vi "Test for renamed Wfms.vi"(4 "Full Path info":bool, 6 "Refresh List":bool, 8 "Error In":errorcluster, 9 "ListBox Variant":variant, 10 "CD Settings":T1={"CD Task Dependency"=18446744073709551615, "CD Task Dependency Ref"=18446744073709551615, "CD Task Available Wfms"=[], "CD Task Selected Wfms"=[], "Buffer Length (samples)"=0, "Min Enabled"=FALSE, "Max Enabled "=FALSE, "SP Enabled"=FALSE, "RMS Enabled"=FALSE, "Buffer Length (s)"=0.0, "Task Rate"=0.0, "Number of DAQ Chanels"=0} {"CD Task Dependency Ref" format="%.0x"; "CD Task Dependency" format="%.0x"}, 11 "CustomDevice Ref":T2 format="%.0x") -> (0 "Error Out":errorcluster, 1 "ListBox Variant":variant, 2 "CD Settings out":T1={"CD Task Dependency"=18446744073709551615, "CD Task Dependency Ref"=18446744073709551615, "CD Task Available Wfms"=[], "CD Task Selected Wfms"=[], "Buffer Length (samples)"=0, "Min Enabled"=FALSE, "Max Enabled "=FALSE, "SP Enabled"=FALSE, "RMS Enabled"=FALSE, "Buffer Length (s)"=0.0, "Task Rate"=0.0, "Number of DAQ Chanels"=0} {"CD Task Dependency Ref" format="%.0x"; "CD Task Dependency" format="%.0x"}, 3 "CustomDevice Ref":T2 format="%.0x", 5 "Names to Remove":string[](array[string]))   [LabVIEW 2017, in "Waveform-Processing-Custom-Device System Explorer.lvlib"]
doc: "This application tests for the senerio of when the origional channel name list was modified and an input channel was renamed, the previous names list is provided so that thay can be removed from the Veristand project. \n\nThis application will also change the name from the full path channel name to the \"user provided\" chanel name."
uses:
  Waveform-Processing-Custom-Device System Explorer.lvlib
  <vilib>/NI Veristand/Custom Device API/Custom Device Item Ref.ctl
  Shared/Custom Device Settings.ctl
  NationalInstruments.VeriStand.SystemStorage
  NationalInstruments.VeriStand
  <userlib>/_OpenG.lib/array/array.llb/Remove Duplicates from 1D Array (String)__ogtk.vi
  <vilib>/NI VeriStand/Custom Device Tools/Custom Device Utility Library/Custom Device Utility Library.lvlib
  <vilib>/NI Veristand/Custom Device API/Custom Device API.lvlib
  Shared/Waveform-Processing-Custom-Device Shared.lvlib
panel:
  out "Number of DAQ Channels":i32 caption="# Ch's"
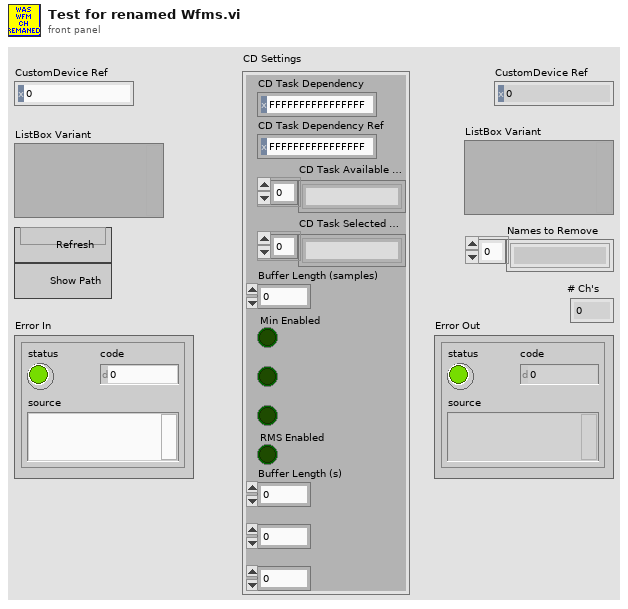
[diagram p1: front panel]
types:
  T1 = typedef "Waveform-Processing-Custom-Device Shared.lvlib/Custom Device Settings.ctl" = cluster{"CD Task Dependency":T2, "CD Task Dependency Ref":T2, "CD Task Available Wfms":string[], "CD Task Selected Wfms":string[], "Buffer Length (samples)":u32, "Min Enabled":bool, "Max Enabled ":bool, "SP Enabled":bool, "RMS Enabled":bool, "Buffer Length (s)":dbl, "Task Rate":dbl, "Number of DAQ Chanels":u32}
  T2 = typedef "Custom Device API.lvlib/Custom Device Item Ref.ctl" = u64
  T3 = typedef "Custom Device API.lvlib/Custom Device Pointer.ctl" = refnum<k24>
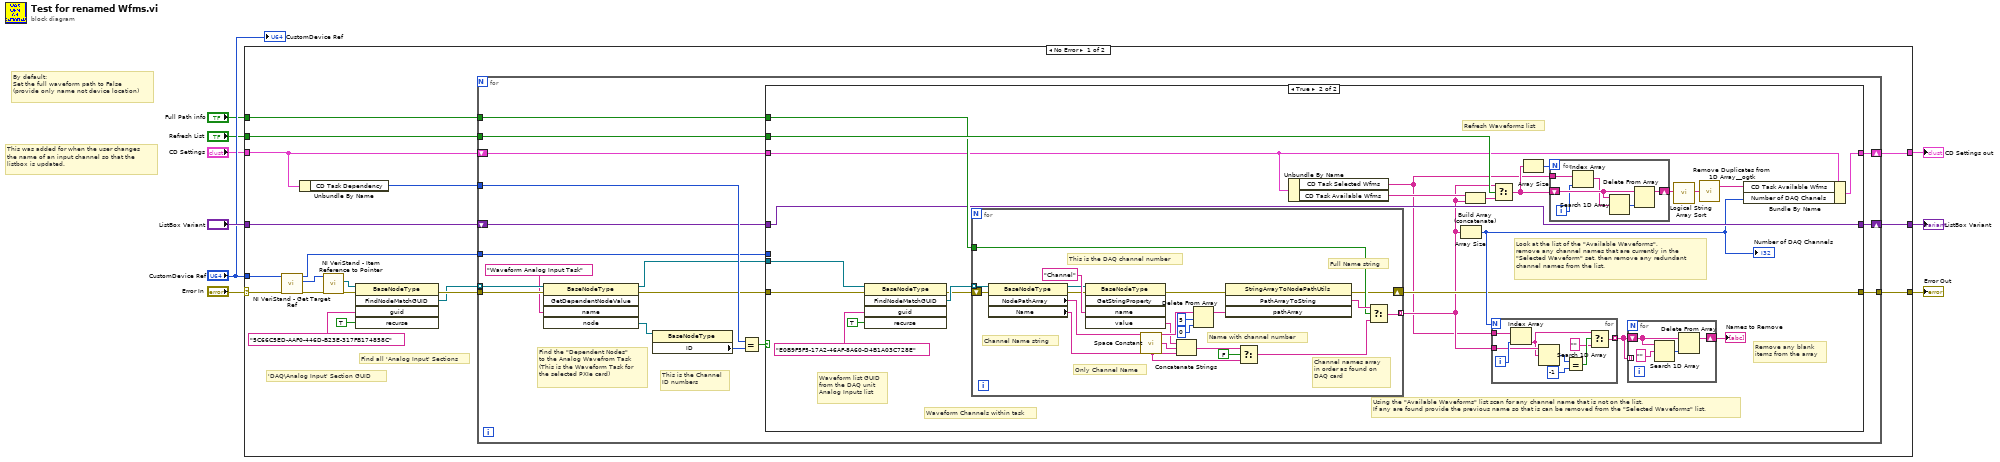
[diagram p0: block diagram]
diagram:
  # "This was added for when the user changes \nthe name of an input channel so that the \nlistbox is updated."
  # "By default:\nSet the full waveform path to False \n(provide only name not device location)"
  n1 = case shown="No Error" "Error In" {
    selector: "Error In" -> [w28 w114]
    tunnel: [w20 w114] -> w4
    tunnel: "CustomDevice Ref" -> [w17 _]
    tunnel: [w19 w113] -> w8
    tunnel: "ListBox Variant" -> [w18 w113]
    tunnel: "CD Settings" -> [w14 w112]
    tunnel: [w13 w112] -> w5
    tunnel: "Refresh List" -> [w11 _]
    tunnel: "Full Path info" -> [w10 _]
    frame No Error {
      # "'DAQ\\Analog Input' Section GUID"
      # "Find all 'Analog Input' Sections"
      n2 = call <vilib>:"NI VeriStand - Get Target Ref.vi"("error in"=w28, "Item Ref in"=w17) -> ("error out"=w27:errorcluster, "Target Ref"=w26:T2, "Item Ref out"=w16:T2)  [unwired: 6 in, 1 out]
      n3 = Unbundle By Name(w14) -> ("CD Task Dependency"=w15:T2)
      n4 = call <vilib>:"NI VeriStand - Item Reference to Pointer.vi"("error in (no error)"=w27, "Item Ref in"=w26) -> ("error out"=w24:errorcluster, "Node Pointer"=w25:T3)  [unwired: 6 in, 2 out]
      n5 = invoke class="BaseNodeType" method="FindNodeMatchGUID"(reference=w25, error in=w24, "guid"="5C66C5ED-AAF0-446D-B23E-317FB174858C" ("Item GUID"), "recurse"=TRUE ("Find All? (T)")) -> (error out=w21:errorcluster, "FindNodeMatchGUID"=w12:refnum<k24>[])  [unwired: 1 in, 3 out]
      n6 = for {
        tunnel: w15 -> [w45]
        tunnel: w12 -> [w44] mode=indexing
        tunnel: w21 -> [w43]
        tunnel: [w38] -> w20
        shift-right: [w37] -> w19
        shift-left: w18 -> [w36]
        tunnel: w16 -> [w35]
        shift-right: [w31] -> w13
        shift-left: w14 -> [w32]
        tunnel: w11 -> [w30]
        tunnel: w10 -> [w29]
        # "This is the Channel\nID numbers"
        # "Find the \"Dependent Nodes\" \nto the Analog Wavefrom Task\n(This is the Waveform Task for \nthe selected PXIe card)"
        n7 = invoke class="BaseNodeType" method="GetDependentNodeValue"(reference=w44, error in=w43, "name"="Waveform Analog Input Task" ("Property Name")) -> (reference out=w33:refnum<k24>, error out=w40:errorcluster, "node"=w34:refnum<k24>)  [unwired: 2 in, 2 out]
        n8 = property class="BaseNodeType"(reference=w34) -> ("ID"=w41:u64)  [unwired: 1 in, 2 out]
        n9 = Equal?(x=w45, y=w41) -> (x = y?=w39:bool)
        n10 = case shown="True" w39 {
          tunnel: w40 -> [w48 w67]
          tunnel: [w48 w51] -> w38
          tunnel: [w47 w55] -> w37
          tunnel: w36 -> [w47 w55]
          tunnel: w35 -> [_ _]
          tunnel: w33 -> [_ w68]
          tunnel: w32 -> [w46 w56]
          tunnel: [w46 w65] -> w31
          tunnel: w30 -> [_ w63]
          tunnel: w29 -> [_ w62]
          frame False {
          }
          frame True {
            # "Remove any blank \nitems from the array"
            # "Using the \"Available Waveforms\" list scan for any channel name that is not on the list. \nIf any are found provide the previous name so that is can be removed from the \"Selected Waveforms\" list."
            # "Refresh Waveforms list"
            # "Look at the list of the \"Available Waveforms\", \nremove any channel names that are currently in the \n\"Selected Waveform\" set, then remove any redundant \nchannel names from the list."
            # "Waveform list GUID\nfrom the DAQ unit\nAnalog Inputs list"
            # "Waveform Channels within task"
            n11 = invoke class="BaseNodeType" method="FindNodeMatchGUID"(reference=w68, error in=w67, "guid"="E0B9F5F5-17A2-46AF-8A60-D4B1A03C728E", "recurse"=TRUE ("Find All? (T)")) -> (error out=w69:errorcluster, "FindNodeMatchGUID"=w70:refnum<k24>[])  [unwired: 1 in, 3 out]
            n12 = for {
              tunnel: w70 -> [w89] mode=indexing
              shift-right: [w74] -> w51
              shift-left: w69 -> [w88]
              tunnel: [w73] -> w50 mode=indexing
              tunnel: w62 -> [w85]
              (unwired) "Channel" ("name")
              # "Channel names array \nin order as found on \nDAQ card"
              # "Only Channel Name"
              # "Name with channel number"
              # "This is the DAQ channel number"
              # "Channel Name string"
              # "Full Name string"
              n13 = property class="BaseNodeType"(reference=w89, error in=w88) -> (reference out=w75:refnum<k24>, error out=w83:errorcluster, "NodePathArray"=w90:string[], "Name"=w76:string)
              n14 = invoke class="BaseNodeType" method="GetStringProperty"(reference=w75, error in=w83, "name"="Channel") -> (error out=w82:errorcluster, "value"=w80:string)  [unwired: 2 in, 3 out]
              n15 = call <vilib>:"Space Constant.vi"() -> ("String"=w81:string)
              n16 = Concatenate Strings(w80, w81, w76) -> (w78:string)
              n17 = Delete From Array(array=w90, length=5, index=0) -> (array with subset deleted=w87:string[])  [unwired: 1 out]
              n18 = invoke class="StringArrayToNodePathUtils" method="PathArrayToString"(error in=w82, "pathArray"=w87) -> (error out=w74:errorcluster, "PathArrayToString"=w86:string)  [unwired: 2 in, 2 out]
              n19 = Select(t=w78, s=FALSE, f=w76) -> (s? t:f=w77:string)
              n20 = Select(t=w86, s=w85, f=w77) -> (s? t:f=w73:string)
            }
            n21 = Unbundle By Name(w56) -> ("CD Task Selected Wfms"=w49:string[], "CD Task Available Wfms"=w66:string[])
            n22 = Array Size(array=w50) -> (size(s)=w52:i32)
            "Number of DAQ Channels" <- w52
            n23 = Build Array (concatenate)(w66, w50) -> (w64:string[])
            n24 = for {
              N: w52 -> [_]
              tunnel: w49 -> [w102]
              tunnel: w50 -> [w100]
              tunnel: [w104] -> w53 mode=indexing
              i -> [w101]
              n25 = Index Array(array=w102, index=w101) -> (element=w99:string)
              n26 = Search 1D Array(1D array=w100, element=w99) -> (index of element=w98:i32)  [unwired: 1 in]
              n27 = Equal?(x=w98, y=-1) -> (x = y?=w105:bool)
              n28 = Select(t=w99, s=w105, f="") -> (s? t:f=w104:string)
            }
            n29 = Select(t=w50, s=w63, f=w64) -> (s? t:f=w61:string[])
            n30 = Array Size(array=w61) -> (size(s)=w60:i32)
            n31 = for {
              N: w60 -> [_]
              tunnel: w49 -> [w110]
              shift-right: [w108] -> w58
              shift-left: w61 -> [w111]
              i -> [w106]
              n32 = Index Array(array=w110, index=w106) -> (element=w107:string)
              n33 = Search 1D Array(1D array=w111, element=w107) -> (index of element=w109:i32)  [unwired: 1 in]
              n34 = Delete From Array(array=w111, index=w109) -> (array with subset deleted=w108:string[])  [unwired: 1 in, 1 out]
            }
            n35 = for {
              shift-right: [w93] -> w54
              shift-left: w53 -> [w96]
              tunnel: w53 -> [_] mode=indexing
              n36 = Search 1D Array(1D array=w96, element="" ("f")) -> (index of element=w95:i32)  [unwired: 1 in]
              n37 = Delete From Array(array=w96, index=w95) -> (array with subset deleted=w93:string[])  [unwired: 1 in, 1 out]
            }
            "Names to Remove" <- w54
            n38 = call "Logical String Array Sort.vi"("Unsorted List"=w58) -> ("Sorted List"=w59:string[])  [unwired: 18 in]
            n39 = call-poly <userlib>:"Remove Duplicates from 1D Array__ogtk.vi"("Input Array"=w59) -> ("Output Array"=w57:string[])  [unwired: 1 out]
            n40 = Bundle By Name(cluster=w56, "CD Task Available Wfms"=w57, "Number of DAQ Chanels"=w52) -> (w65:T1)
          }
        }
      }
    }
    frame Error {
    }
  }
  "ListBox Variant" <- w8
  "CD Settings out" <- w5
  "Error Out" <- w4
  "CustomDevice Ref" <- "CustomDevice Ref"
